vi "Proceed own msg.vi"(9 "priority":i32, 10 "Proxy.lvlib:Proxy Msg Base.lvclass":refnum<class "Proxy Msg Base.lvclass">, 11 "Proxy in":refnum<class "Proxy.lvclass">) -> (0 "error out":errorcluster, 3 "Actor out":refnum<class "Actor.lvclass">)   [LabVIEW 2014, in "Proxy.lvlib" / "Proxy.lvclass"]
uses:
  Proxy.lvclass
  Proxy Msg Base/Proxy Msg Base.lvclass
  <vilib>/ActorFramework/Actor/Actor.lvclass
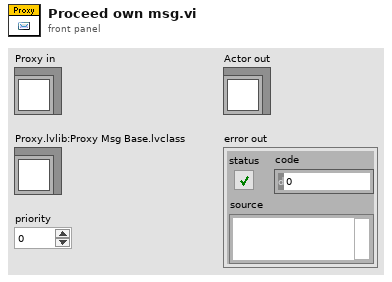
[diagram p1: front panel]
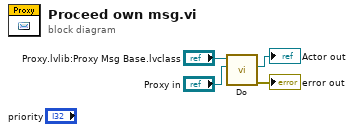
[diagram p0: block diagram]
diagram:
  n1 = call-dynamic "Do.vi"("Actor in"="Proxy in", "Message"="Proxy.lvlib:Proxy Msg Base.lvclass") -> ("error out"=→"error out":errorcluster, "Actor out"=→"Actor out":refnum<class "Actor.lvclass">)  [unwired: 8 in]
